vi "Set Tiles Info.vi"(8 "error in (no error)":errorcluster, 10 "Tiles Info":string[][](array[string]), 11 "Tiles Info Msg in":refnum<class "Tiles Info Msg.lvclass">) -> (0 "error out":errorcluster, 3 "Tiles Info Msg out":refnum<class "Tiles Info Msg.lvclass">)   [LabVIEW 2013, in "Project Model.lvlib" / "Tiles Info Msg.lvclass"]
uses:
  Tiles Info Msg.lvclass
  Tiles Info Msg.lvclass/Tiles Info Msg.ctl
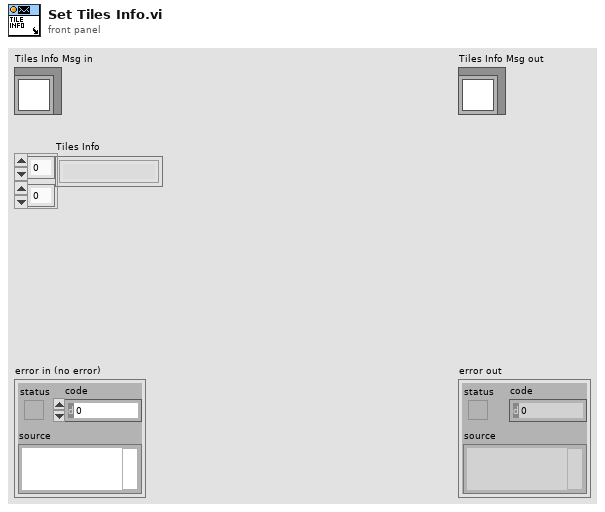
[diagram p1: front panel]
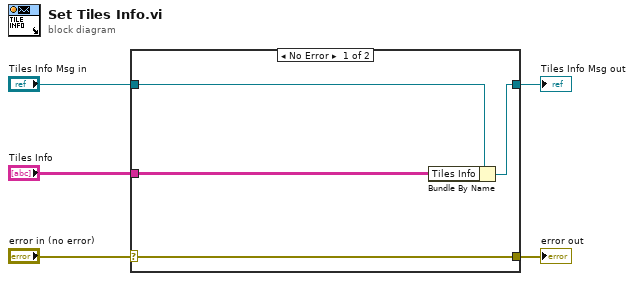
[diagram p0: block diagram]
diagram:
  n1 = case shown="No Error" "error in (no error)" {
    selector: "error in (no error)" -> [w9 w10]
    tunnel: [w9 w10] -> w4
    tunnel: [w7 w11] -> w2
    tunnel: "Tiles Info Msg in" -> [w8 w11]
    tunnel: "Tiles Info" -> [w6 _]
    frame No Error {
      n2 = Bundle By Name(cluster=w8, "Tiles Info"=w6) -> (w7:refnum<class "Tiles Info Msg.lvclass">)
    }
    frame Error {
    }
  }
  "error out" <- w4
  "Tiles Info Msg out" <- w2
